vi "TestNeutronDetector.vi"() -> ()   [LabVIEW 2018]
panel:
  out "data":dbl
  in  "stop (F)":bool
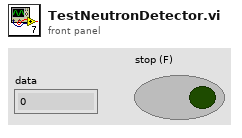
[diagram p1: front panel]
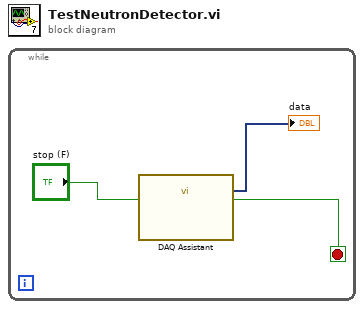
[diagram p0: block diagram]
diagram:
  n1 = while {
    stop <- w3 stop-if-true
    n2 = call "DAQ Assistant"("stop (F)"="stop (F)") -> ("data"=→"data":dynamicdata, "stopped"=w3:bool)  [unwired: 15 in, 2 out]
  }
